vi "DecayRateShaken.vi"() -> ()   [LabVIEW 2015]
uses:
  <vilib>/Utility/file.llb/Read Delimited Spreadsheet (DBL).vi
panel:
  out "Decay Plot":dbl[][](graph)
  in  "Shaken Water":path=path "C:/Users/Brian/Desktop/New folder/week8/Unshaken_Water"
  out "Decay Time":dbl
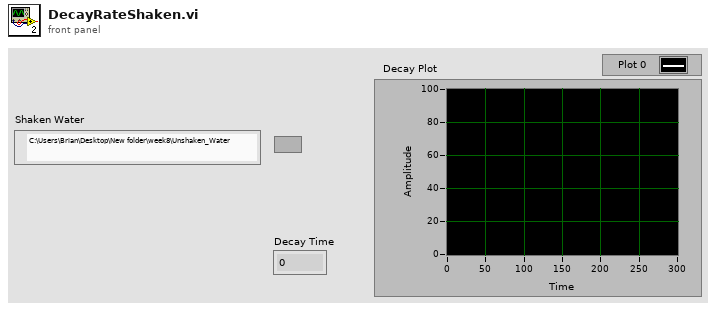
[diagram p1: front panel]
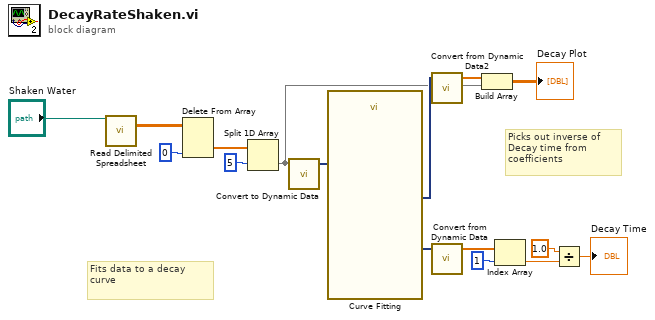
[diagram p0: block diagram]
diagram:
  # "Picks out inverse of Decay time from coefficients"
  # "Fits data to a decay curve"
  n1 = call-poly <vilib>:"Read Delimited Spreadsheet.vi"("file path (dialog if empty)"="Shaken Water") -> ("all rows"=w6:dbl[][])  [unwired: 9 in, 5 out]
  n2 = Delete From Array(array=w6, index (col)=0) -> (deleted portion=w8:dbl[])  [unwired: 2 in, 1 out]
  n3 = Split 1D Array(array=w8, index=5) -> (second subarray=w3:dbl[])  [unwired: 1 out]
  n4 = call "Convert to Dynamic Data"("Array"=w3) -> ("Dynamic Data Type"=w16:dynamicdata)  [unwired: 3 in]
  n5 = call "Curve Fitting"("Signals"=w16) -> ("best fit"=w4:dynamicdata, "non-linear coefficients"=w15:dynamicdata)  [unwired: 6 in, 3 out]
  n6 = call "Convert from Dynamic Data2"("Dynamic Data Type"=w4) -> ("Array"=w2:dbl[])  [unwired: 3 in]
  n7 = call "Convert from Dynamic Data"("Dynamic Data Type"=w15) -> ("Array"=w14:dbl[])  [unwired: 3 in]
  n8 = Build Array(w2, w3) -> (→"Decay Plot":dbl[][])
  n9 = Index Array(array=w14, index=1) -> (element=w12:dbl)
  n10 = Divide(x=1.0, y=w12) -> (x/y=→"Decay Time":dbl)
